vi "05-QNET_MECHKIT_Infrared.vi"() -> ()   [LabVIEW 2017]
doc: "This VI is to be used with the NI-ELVIS and the QNET-Mechatronic Sensors I module. The objective is to calibrate the infrared sensor."
uses:
  <vilib>/Simulation/Scripting/Companion Diagram/SimConfigNode/SimParams.ctl
  <vilib>/Simulation/Scripting/Companion Diagram/SimConfigNode/_simSolvers.ctl
  <vilib>/Simulation/Implementation/Shared/SIMSCR Execution Mode.ctl
  <vilib>/Simulation/Param Hierarchy/Typedefs/SIMPH Param Control Actions.ctl
  <vilib>/Simulation/Implementation/Shared/NILVSim_ParamChanged.vi
  <vilib>/Simulation/Implementation/Shared/NILVSIM_BeginStep.vi
  <vilib>/DAQmx/read.llb/DAQmx Read.vi
  <vilib>/DAQmx/read.llb/DAQmx Read (Analog DBL 1Chan 1Samp).vi
  <vilib>/Simulation/SignalDisplay/Implementation/NILVSim Time Waveform.llb/SIM Time Waveform (scalar).vi
  <vilib>/Simulation/Utility/Implementation/SIM Halt.vi
  <vilib>/Simulation/Implementation/Shared/NILVSim_Manager.vi
  <vilib>/Utility/error.llb/Clear Errors.vi
  <vilib>/Simulation/Implementation/Shared/NILVSim_FinalizeModel.vi
  <vilib>/Simulation/Implementation/Shared/SIM Unbundle Sim Info.vi
  <vilib>/Simulation/Implementation/Shared/NILVSim_Initialize.vi
  <vilib>/Analysis/6fits.llb/General Polynomial Fit.vi
  <vilib>/DAQmx/miscellaneous.llb/DAQmx Fill In Error Info.vi
  <vilib>/Simulation/Utility/Implementation/NILVSim Get Time and IsAcceptedStep.vi
  <vilib>/Simulation/Implementation/Shared/SIMSH Read Queue.vi
  <vilib>/Simulation/Implementation/Shared/NILVSim_GetModelError.vi
  <vilib>/Simulation/Implementation/Shared/SIM Bundle Sim Info.vi
  <vilib>/Simulation/Scripting/Companion Diagram/SimConfigNode/SimDog.xnode
  <vilib>/Simulation/Implementation/XNodeFramework/SimXNode/SimX.xnode
  <vilib>/Analysis/NI_AALPro.lvlib
  <vilib>/Simulation/Implementation/Shared/NI_SIM_Implementation.lvlib
panel:
  in  "Sampling Rate (Hz)":dbl=100.0 min=0.0 max=1000.0 step=25.0 format="%.1f"
  in  "Device":tag="Dev1"
  in  "Tab Control":enum32{"Collect Data", "Calibrate Sensor"}(tab)
  out "Infrared Sensor (V)":waveform(dbl)(graph)
  in  "Target Range (cm)":dbl[](array[numeric])
  in  "Sensor Measurement (V)":dbl[](array[numeric])
  out "Sensor Readings":T1(graph)
  out "Coefficients: y = a*x^2 + b*x + c":dbl[](array[numeric]) format="%0.2f"
  out "IR (cm)":dbl(knob) scale=0.0..100.0
  in  "c (cm)":dbl
  in  "a (cm/V^2)":dbl
  out "IR Sensor (cm)":waveform(dbl)(graph)
  in  "b (cm/V)":dbl
  in  "stop":bool
  # "QNET-MECHKIT Infrared Sensor"
  # "NOTE 1: Place J10 jumper on \"Infrared\" setting.\nNOTE 2: Turn on the IR switch. The \"IR ON\" LED should be bright red."
  # "1) Move target at different positions.\n2) Enter distance between IR and target in \"Target Position (cm)\" array.\n3) Enter measured sensor values in \"Sensor Measurement (V)\" array."
  # "Polynomial curve fitting results:"
  # "c"
  # "b"
  # "a"
  # "Enter polynomial coefficients to measure correct target distance \n(e.g. display below should read 25.0 cm when target is 25.0 cm away from IR sensor)."
  # "y = a*x^2 + b*x + c\nwhere\nx is the sensor voltage \ny is the output in centimeters."
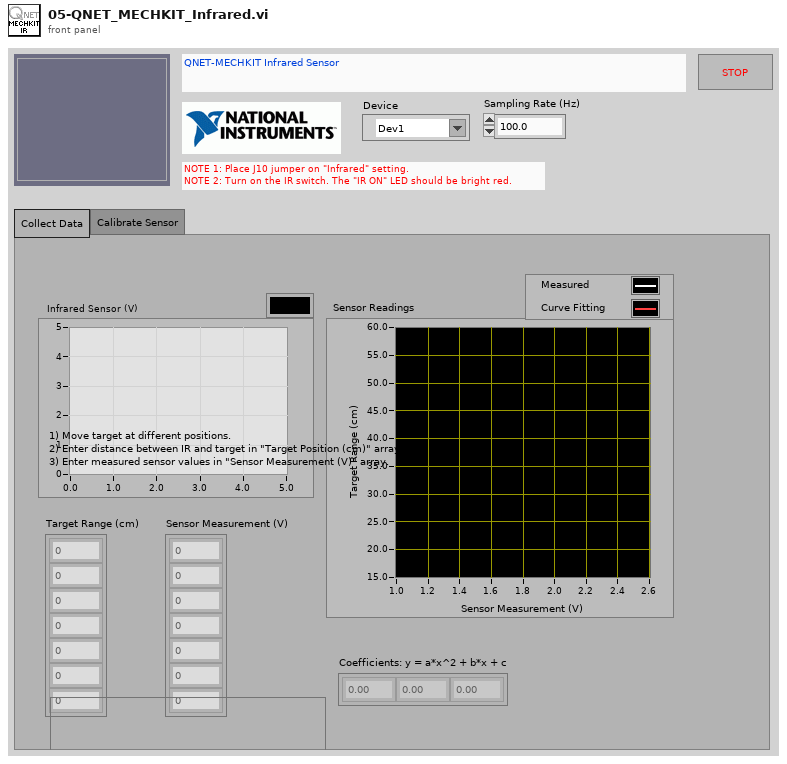
[diagram p1: front panel]
types:
  T1 = cluster{"Sensor Measurement (V)":dbl[], "Best Linear Fit":dbl[]}[]
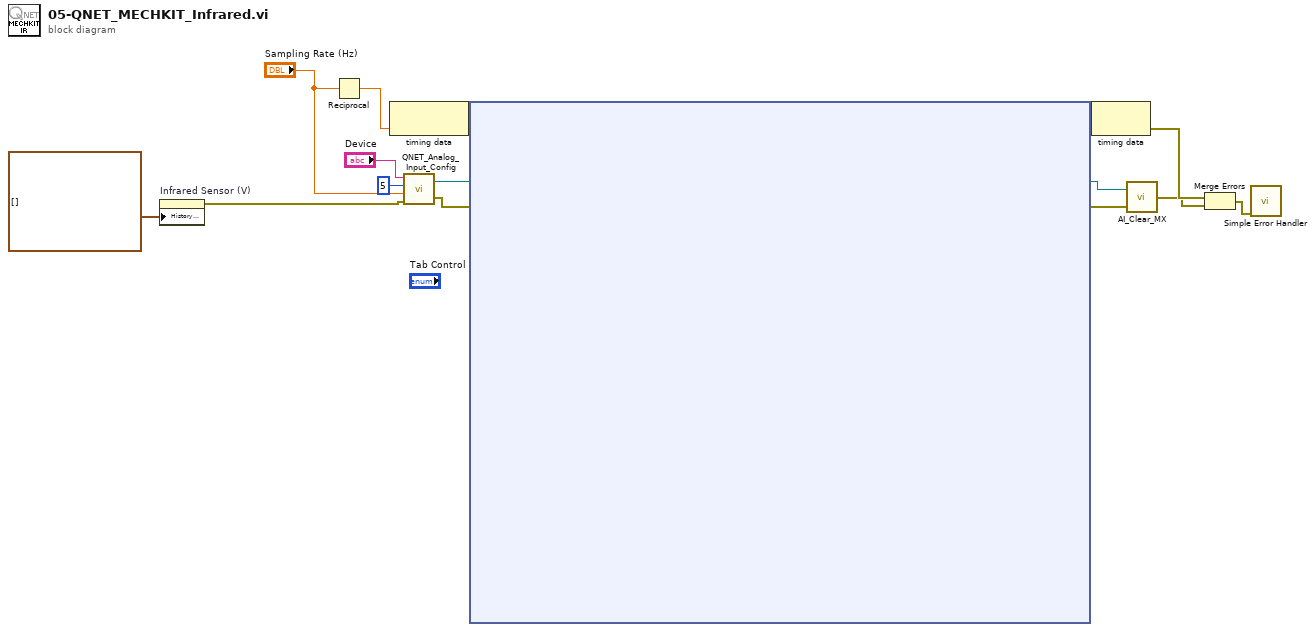
[diagram p0: block diagram]
diagram:
  n1 = property on="Infrared Sensor (V)" class="WFChart (strict)"("History Data"=waveform(dbl)[] []) -> (error out=w2:errorcluster)  [unwired: 2 in, 1 out]
  n2 = Reciprocal(x="Sampling Rate (Hz)") -> (1/x=w6:dbl)
  n3 = node-c288(w6) -> (w14:variant)
  n4 = call "QNET_Analog_Input_Config.vi"("error in"=w2, "sampling rate (Hz)"="Sampling Rate (Hz)", "analog input channel"=u32 5, "dev"="Device") -> ("error out"=w11:errorcluster, "task out"=w10:refnum<k21>)
  n5 = node-c254 ("Simulation Loop")(w14, w11, w10) -> (w13:variant, w9:refnum<k21>, w8:errorcluster)
  n6 = node-c288(w13) -> (w5:errorcluster)
  n7 = call "AI_Clear_MX.vi"("Error in"=w8, "Task in"=w9) -> ("Error out"=w4:errorcluster)
  n8 = Merge Errors(w5, w4) -> (w3:errorcluster)
  n9 = call <vilib>:"Simple Error Handler.vi"("error in (no error)"=w3) -> ()  [unwired: 1 in, 8 out]
